vi "SetShutters.vi"(8 "error in (no error)":errorcluster, 10 "Shutters":T1, 11 "Operational Mode":T4) -> (0 "error out":errorcluster, 2 "Shutters out":T1, 3 "Operational Mode out":T4)   [LabVIEW 2016]
uses:
  Controls/Operational Modes.ctl
  Controls/Shutters.ctl
  Controls/Shutter Data.ctl
  Controls/Shutter States.ctl
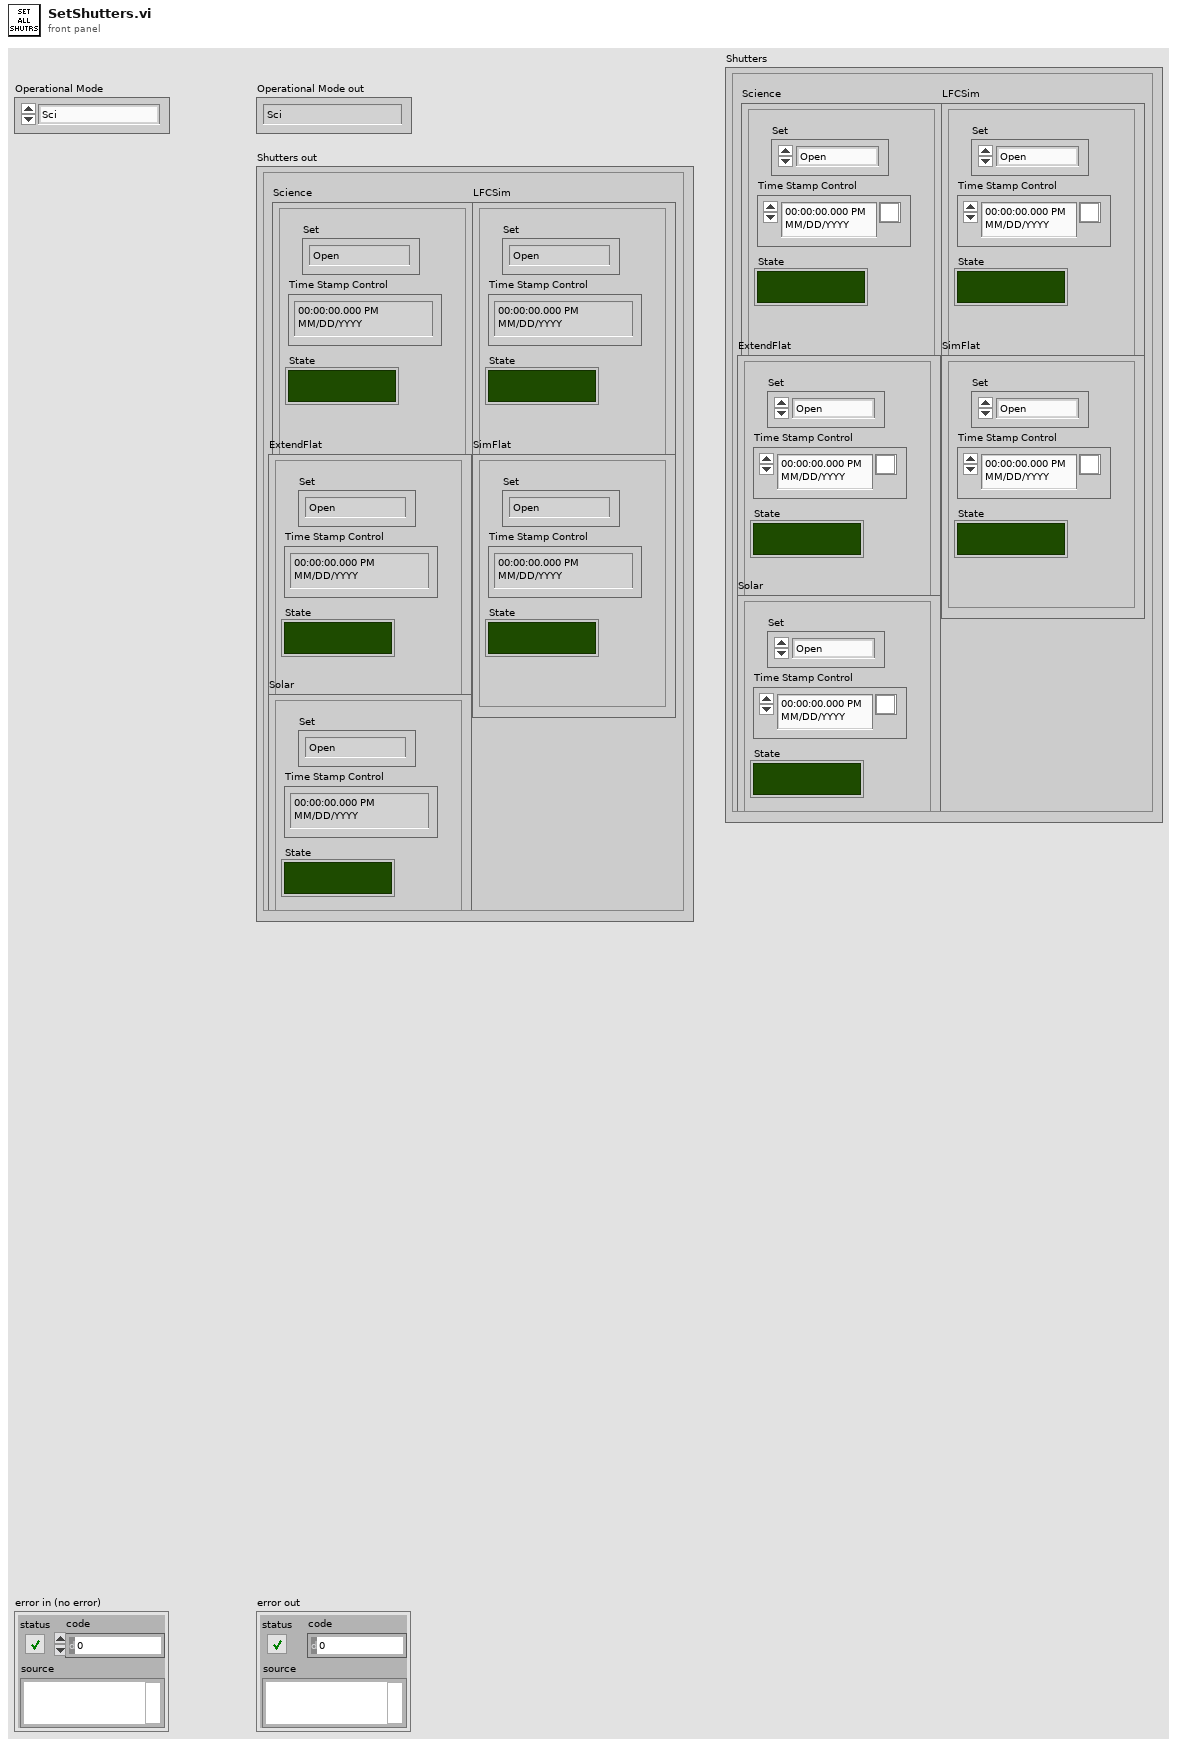
[diagram p1: front panel]
types:
  T1 = typedef "Shutters.ctl" = cluster{"Science":T2, "LFCSim":T2, "ExtendFlat":T2, "SimFlat":T2, "Solar":T2}
  T2 = typedef "Shutter Data.ctl" = cluster{"Time Stamp Control":timestamp, "State":bool, "Set":T3}
  T3 = typedef "Shutter States.ctl" = enum16{"Open", "Close", "Wait", "Off", "Arm", "Idle"}
  T4 = typedef "Operational Modes.ctl" = enum16{"Sci", "Sci-LFC", "Solar", "Solar-LFC", "LFC", "LFC-Sim", "LFC-Both", "ThAr", "ThAr-LFC", "Flat", "ExtFlat", "ExtFlat-Sim", "ExtFlat-Both", "Qtz", "ExtQtz", "ExtQtz-Sim", "ExtQtz-Both", "Dark", "Manual", "Off"}
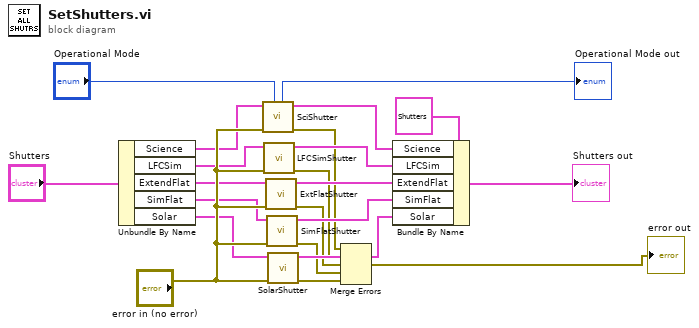
[diagram p0: block diagram]
diagram:
  n1 = Unbundle By Name("Shutters") -> ("Science"=w4:T2, "LFCSim"=w6:T2, "ExtendFlat"=w7:T2, "SimFlat"=w8:T2, "Solar"=w9:T2)
  n2 = call "SciShutter.vi"("Operational Mode"="Operational Mode", "error in (no error)"="error in (no error)", "Science"=w4) -> ("error out"=w10:errorcluster, "Science out"=w15:T2, "Operational Mode out"=→"Operational Mode out":T4)  [unwired: 6 in]
  n3 = call "LFCSimShutter.vi"("error in (no error)"="error in (no error)", "LFCSim"=w6) -> ("error out"=w11:errorcluster, "LFCSim out"=w16:T2)  [unwired: 8 in]
  n4 = call "ExtFlatShutter.vi"("error in (no error)"="error in (no error)", "ExtFlat"=w7) -> ("error out"=w12:errorcluster, "ExtFlat out"=w18:T2)  [unwired: 8 in]
  n5 = call "SimFlatShutter.vi"("error in (no error)"="error in (no error)", "SimFlat"=w8) -> ("error out"=w13:errorcluster, "SimFlat out"=w20:T2)  [unwired: 8 in]
  n6 = call "SolarShutter.vi"("error in (no error)"="error in (no error)", "Solar"=w9) -> ("error out"=w14:errorcluster, "Solar out"=w19:T2)  [unwired: 8 in]
  n7 = Merge Errors(w10, w11, w12, w13, w14) -> (→"error out":errorcluster)
  n8 = Bundle By Name(cluster=T1 {"Science"={"Time Stamp Control"=timestamp(0 s since 1904-01-01), "State"=FALSE, "Set"=enum."Open"}, "LFCSim"={"Time Stamp Control"=timestamp(0 s since 1904-01-01), "State"=FALSE, "Set"=enum."Open"}, "ExtendFlat"={"Time Stamp Control"=timestamp(0 s since 1904-01-01), "State"=FALSE, "Set"=enum."Open"}, "SimFlat"={"Time Stamp Control"=timestamp(0 s since 1904-01-01), "State"=FALSE, "Set"=enum."Open"}, "Solar"={"Time Stamp Control"=timestamp(0 s since 1904-01-01), "State"=FALSE, "Set"=enum."Open"}} ("Shutters"), "Science"=w15, "LFCSim"=w16, "ExtendFlat"=w18, "SimFlat"=w20, "Solar"=w19) -> (→"Shutters out":T1)
